vi "Test Process Context not Set on Upstreams Error.vi"(8 "error in (no error)":errorcluster, 11 "Process Dev Test in":refnum<class "Process Dev Test.lvclass">) -> (0 "error out":errorcluster, 3 "Process Dev Test out":refnum<class "Process Dev Test.lvclass">)   [LabVIEW 2020, in "Process Dev Test.lvclass"]
uses:
  Process Dev Test.lvclass
  C:/Program Files (x86)/National Instruments/LabVIEW 2020/vi.lib/Astemes/LUnit/Test Case.lvclass
  source/Framework/Process/Process.lvclass
  source/Framework Test Suite/Mock Process/Mock Process.lvclass
  C:/Git/triarc-framework/source/Framework/Error Handler Interface/Error Handler Interface.lvclass
  source/Framework/Process/Process.lvclass/Process.ctl
  <vilib>/Astemes/LUnit/Test Case.lvclass/Test Case.ctl
  6b13e907-0495-49fd-9976-d192fb7ff710.vi
  source/Framework/Process/Protected/Messaging/Send Message.vi
  source/Framework/Process/Public/Lifecycle/Get Lifecycle State.vi
  source/Framework/Process/Protected/SubVIs/Set Context.vi
  <vilib>/Astemes/LUnit/Palette/Pass.vi
  <vilib>/Astemes/LUnit/Palette/Fail.vi
  <vilib>/Astemes/LUnit/Compare Variants.vi
  <vilib>/Astemes/LUnit/Describe Comparison.vi
  <vilib>/Astemes/LUnit/Set Assertion Type.vi
  source/Framework/Process/Private/SubVIs/Handle Debug Data.vi
  source/Framework/Process/Public/Lifecycle/Leave Process Loop.vi
  <vilib>/Astemes/LUnit/Add test result.vi
  <vilib>/Astemes/LUnit/Variant to string.vi
  <vilib>/Utility/High Resolution Relative Seconds.vi
  <vilib>/Astemes/LUnit/LUnit Record Assertion Result.vi
  <vilib>/Astemes/LUnit/LUnit Aggregate Assertion Results.vi
  <vilib>/Astemes/LUnit/Method Result/LUnit Merge Status.vi
  <vilib>/Astemes/LUnit/LUnit Concatenate result strings.vi
  <vilib>/Utility/error.llb/Error Cluster From Error Code.vi
  <vilib>/Utility/Data Type/Get Type Information.vi
  <vilib>/Utility/LVClass/Get LV Class Name.vi
panel:
  out "Qualified Name":string
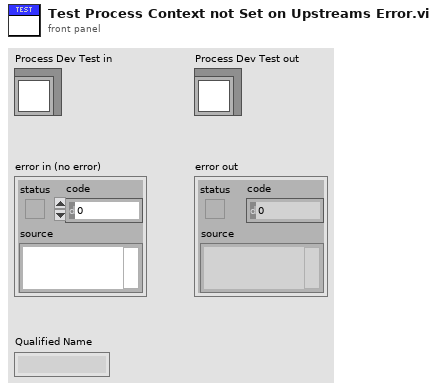
[diagram p1: front panel]
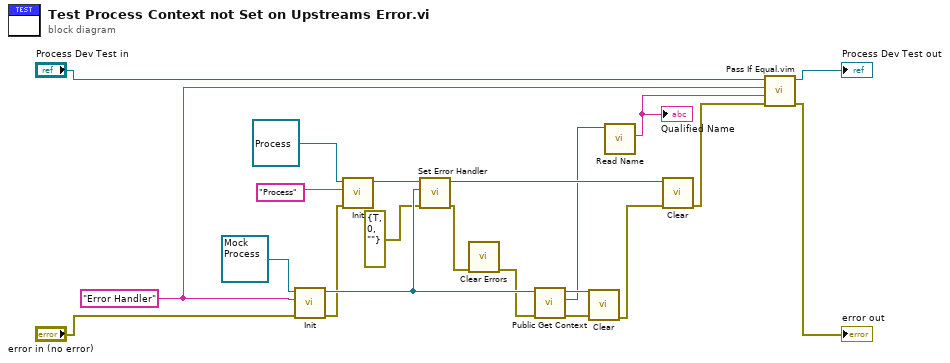
[diagram p0: block diagram]
diagram:
  w1 = "Error Handler" ("Name")
  n1 = call-dynamic "Init.vi"("error in (no error)"="error in (no error)", "Name"=w1, "Mock Process In"=refnum<class "Mock Process.lvclass"> refnum ("Mock Process.lvclass")) -> ("error out"=w12:errorcluster, "Mock Process Out"=w16:refnum<class "Mock Process.lvclass">)  [unwired: 7 in]
  n2 = call-dynamic "Init.vi"("error in (no error)"=w12, "Name"="Process", "Process In"=refnum<class "Process.lvclass"> refnum ("Process.lvclass")) -> ("Process Out"=w19:refnum<class "Process.lvclass">)  [unwired: 7 in, 1 out]
  n3 = call "Set Error Handler.vi"("error in (no error)"=errorcluster {"status"=TRUE, "code"=0, "source"=""}, "Error Handler"=w16, "Process In"=w19) -> ("error out"=w15:errorcluster, "Process Out"=w18:refnum<class "Process.lvclass">)  [unwired: 7 in]
  n4 = call <vilib>:"Clear Errors.vi"("error in (no error)"=w15) -> ("error out"=w2:errorcluster)  [unwired: 5 in, 1 out]
  n5 = call "Public Get Context.vi"("error in (no error)"=w2, "Mock Process in"=w16) -> ("error out"=w17:errorcluster, "Context"=w10:refnum<class "Process.lvclass">, "Mock Process out"=w13:refnum<class "Mock Process.lvclass">)  [unwired: 7 in]
  n6 = call-dynamic "Clear.vi"("error in (no error)"=w17, "Mock Process In"=w13) -> ("error out"=w14:errorcluster)  [unwired: 9 in]
  n7 = call "Read Name.vi"("Process In"=w10) -> ("Qualified Name"=w9:string)  [unwired: 7 in, 3 out]
  "Qualified Name" <- w9
  n8 = call-dynamic "Clear.vi"("error in (no error)"=w14, "Process In"=w18) -> ("error out"=w11:errorcluster)  [unwired: 9 in]
  n9 = call "Pass If Equal.vim"("error in (no error)"=w11, "Actual"=w9, "Expected"=w1, "LUnit Test Case In"="Process Dev Test in") -> ("error out"=→"error out":errorcluster, "LUnit Test Case Out"=→"Process Dev Test out":refnum<class "Process Dev Test.lvclass">)  [unwired: 6 in]
